vi "Update cursors.vi"(8 "error in (no error)":errorcluster, 10 "Cluster in":T1 {"Limit stop" min=0.0 max=150.0 step=0.0001; "Speed" min=0.0001 max=20.0 step=0.0001; "Home pos" min=0.0 max=150.0 step=0.0001}, 11 "LIVE DATA 3":refnum<vi>) -> (0 "error out":errorcluster)   [LabVIEW 2016]
uses:
  Actuator/Controls/Default settings.ctl
  Cursor data.ctl
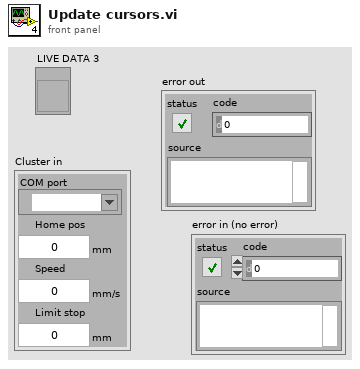
[diagram p1: front panel]
types:
  T1 = typedef "Default settings.ctl" = cluster{"COM port":refnum<visa-resource-name>, "Home pos":dbl, "Speed":dbl, "Limit stop":dbl}
  T2 = cluster{"Name":string, "Color":u32, "Style":u8, "Point Style":u8, "Name Visible":bool, "Allow Drag":bool, "Cursor Mode":u32, "Plot":i32, "Index":i32, "Position":cluster{"X":dbl, "Y":dbl}, "X Scale":u32, "Y Scale":u32, "Watch Plots":i32[], "Watch All Plots":bool, "Plot Area":i32, "Label Offset":cluster{"X":dbl, "Y":dbl}}
  T3 = typedef "Cursor data.ctl" = cluster{"Name":string, "Colour":u32}
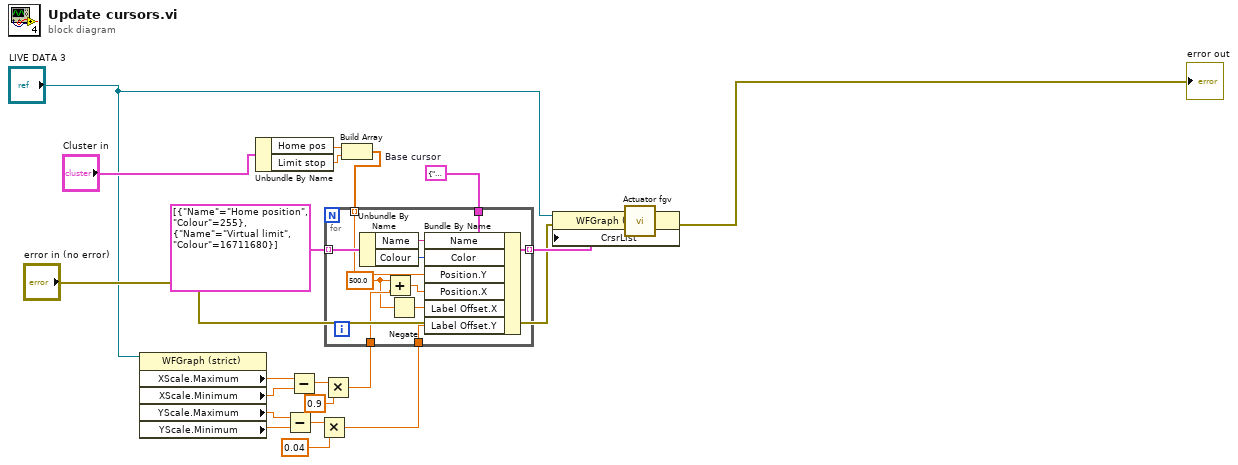
[diagram p0: block diagram]
diagram:
  w14 = T2 {"Name"="", "Color"=0, "Style"=6, "Point Style"=0, "Name Visible"=TRUE, "Allow Drag"=TRUE, "Cursor Mode"=0, "Plot"=0, "Index"=0, "Position"={"X"=0.0, "Y"=0.0}, "X Scale"=0, "Y Scale"=0, "Watch Plots"=[], "Watch All Plots"=FALSE, "Plot Area"=0, "Label Offset"={"X"=0.0, "Y"=0.0}}  # Base cursor
  n1 = property class="WFGraph (strict)"(reference="LIVE DATA 3") -> ("XScale.Maximum"=w11:dbl, "XScale.Minimum"=w10:dbl, "YScale.Maximum"=w6:dbl, "YScale.Minimum"=w5:dbl)  [unwired: 1 in, 2 out]
  n2 = Unbundle By Name("Cluster in") -> ("Home pos"=w18:dbl, "Limit stop"=w19:dbl)
  n3 = Subtract(x=w6, y=w5) -> (x-y=w4:dbl)
  n4 = Subtract(x=w11, y=w10) -> (x-y=w9:dbl)
  n5 = Multiply(x=w4, y=0.04) -> (x*y=w2:dbl)
  n6 = Multiply(x=w9, y=0.9) -> (x*y=w7:dbl)
  n7 = Build Array(w18, w19) -> (w20:dbl[])
  n8 = for {
    tunnel: w14 -> [w31]
    tunnel: [w30] -> w16 mode=indexing
    tunnel: T3[] [{"Name"="Home position", "Colour"=255}, {"Name"="Virtual limit", "Colour"=16711680}] -> [w29] mode=indexing
    tunnel: w20 -> [w26] mode=indexing
    tunnel: w7 -> [w24]
    tunnel: w2 -> [w25]
    w22 = 500.0 ("x")
    n9 = Unbundle By Name(w29) -> ("Name"=w28:string, "Colour"=w27:u32)
    n10 = Add(x=w22, y=w24) -> (x+y=w23:dbl)
    n11 = Negate(x=w22) -> (-x=w21:dbl)
    n12 = Bundle By Name(cluster=w31, "Name"=w28, "Color"=w27, "Position.Y"=w26, "Position.X"=w23, "Label Offset.X"=w21, "Label Offset.Y"=w25) -> (w30:T2)
  }
  n13 = property class="WFGraph (strict)"(reference="LIVE DATA 3", error in="error in (no error)", "CrsrList"=w16) -> (error out=→"error out":errorcluster)  [unwired: 1 out]
  n14 = call "Actuator fgv.vi"() -> ()  [unwired: 10 in, 2 out]
